vi "Memory Throughput Test PXIe-796XR (FPGA).vi"() -> ()   [LabVIEW 2013]
doc: "This test writes to and reads from external memory at maximum data rates and reports the total measured throughput. Varying the write and read grant time will directly affect the memory efficiency. The larger the grant time, then the larger the througput, and the lower the grant time, then the lower the throughput.\n\nDuring reads, the data is validated against an expected pattern. Failures will cause \"Read Data Error?\" to illuminate. To avoid read data errors, a full iteration of memory writes must be completed before starting the memory reads."
uses:
  <vilib>/Platform/TimedLoop/XDataNode/timing_clust.ctl
  <vilib>/Platform/TimedLoop/XDataNode/nitl_modes.ctl
  <vilib>/Platform/TimedLoop/XDataNode/wakeup.ctl
  DRAMElemReaderState.ctl
  Read Request Command.ctl
  <vilib>/rvi/Emulation/niFpgaSctlEmulationGetInTimedLoop.vi
  <vilib>/rvi/Emulation/niFpgaEmulationReportErrorSimple.vi
  <vilib>/rvi/Emulation/niFpgaGetClockAttributes.vi
  <vilib>/rvi/Emulation/niFpgaCriticalErrorInLSC.vi
  <vilib>/rvi/FIFO/Fifo_Resource/nirvififoEmulationWriteFpgaImpl.vi
  <vilib>/rvi/DataTransferAndStorage/Container/Common/niFpgaContainerGetUniqueNameForEmu.vi
  <vilib>/rvi/FIFO/Fifo_Resource/nirvififoEmulationReadFpgaImpl.vi
  <vilib>/rvi/Memory/Memory_Emulation/niFpgaMemoryEmulationReadFromVariant.vi
  <vilib>/rvi/Memory/Memory_Emulation/niFpgaMemoryFastEmulationDramWriteAndRequestData.vi
  <vilib>/rvi/Memory/Memory_Emulation/niFpgaMemoryEmulationDramWriteAndRequestData.vi
  <vilib>/rvi/Memory/Memory_Emulation/niFpgaMemoryEmulationWriteToVariant.vi
  <vilib>/Platform/TimedLoop/XDataNode/XDataNode.xnode
  <vilib>/rvi/DataTransferAndStorage/Container/XNode/niFpgaContainer.xnode
  <vilib>/rvi/FIFO/Fifo_Resource/nirvififoEmulationWrite.vi
  <vilib>/rvi/FIFO/Fifo_Resource/nirvififoEmulationRead.vi
  <vilib>/rvi/Memory/Memory_Emulation/niFpgaMemoryEmulationDramRetrieveData.vi
  <vilib>/Platform/TimedLoop/XDataNode/XDNodeRunTimeDep.lvlib
panel:
  in  "Write Req Grant Time (Bank 1)":u16=1000 caption="Write Req Grant Time (clocks)"
  in  "Read Req Grant Time (Bank 1)":u16=1000 caption="Read Req Grant Time (clocks)"
  in  "Read Req Grant Time (Bank 0)":u16=1000 caption="Read Req Grant Time (clocks)"
  in  "Write Req Grant Time (Bank 0)":u16=1000 caption="Write Req Grant Time (clocks)"
  out "Current Write Data Lower (Bank 0)":u64 caption="Current Write Data Lower" format="%.0x"
  out "Current Write Data Upper (Bank 0)":u64 caption="Current Write Data Upper" format="%.0x"
  out "Current Write Data Lower (Bank 1)":u64 caption="Current Write Data Lower" format="%.0x"
  out "Current Read Data Lower (Bank 1)":u64 caption="Current Read Data Lower" format="%.0x"
  out "Current Read Data Lower (Bank 0)":u64 caption="Current Read Data Lower" format="%.0x"
  out "Current Write Data Upper (Bank 1)":u64 caption="Current Write Data Upper" format="%.0x"
  out "Current Write Address (Bank 1)":u32 caption="Current Write Address" format="%.0x"
  in  "Enable Writes? (Bank 1)":bool=TRUE caption="Enable Writes?"
  out "Write Throughput (bytes/sec) (Bank 1)":u32 caption="Write Throughput (bytes/sec)" format="%.2e"
  out "Read FIFO Overflow? (Bank 1)":bool caption="Read FIFO Overflow?"
  out "Read Data Error? (Bank 1)":bool caption="Read Data Error?"
  out "Current Read Data Upper (Bank 1)":u64 caption="Current Read Data Upper" format="%.0x"
  out "Current Read Address (Bank 1)":u32 caption="Current Read Address" format="%.0x"
  in  "Enable Reads? (Bank 1)":bool caption="Enable Reads?"
  out "Read Throughput (bytes/sec) (Bank 1)":u32 caption="Read Throughput (bytes/sec)" format="%.2e"
  in  "DRAM Size (elements) (Bank 1)":u32=16777216 caption="DRAM Size (elements)"
  out "Read Data Error? (Bank 0)":bool caption="Read Data Error?"
  out "Write Throughput (bytes/sec) (Bank 0)":u32 caption="Write Throughput (bytes/sec)" format="%.2e"
  out "Read Throughput (bytes/sec) (Bank 0)":u32 caption="Read Throughput (bytes/sec)" format="%.2e"
  in  "Enable Reads? (Bank 0)":bool caption="Enable Reads?"
  out "Read FIFO Overflow? (Bank 0)":bool caption="Read FIFO Overflow?"
  in  "Enable Writes? (Bank 0)":bool=TRUE caption="Enable Writes?"
  out "Current Read Data Upper (Bank 0)":u64 caption="Current Read Data Upper" format="%.0x"
  in  "DRAM Size (elements) (Bank 0)":u32=16777216 caption="DRAM Size (elements)"
  out "Current Read Address (Bank 0)":u32 caption="Current Read Address" format="%.0x"
  out "Current Write Address (Bank 0)":u32 caption="Current Write Address" format="%.0x"
  # "Bank 0"
  # "Bank 1"
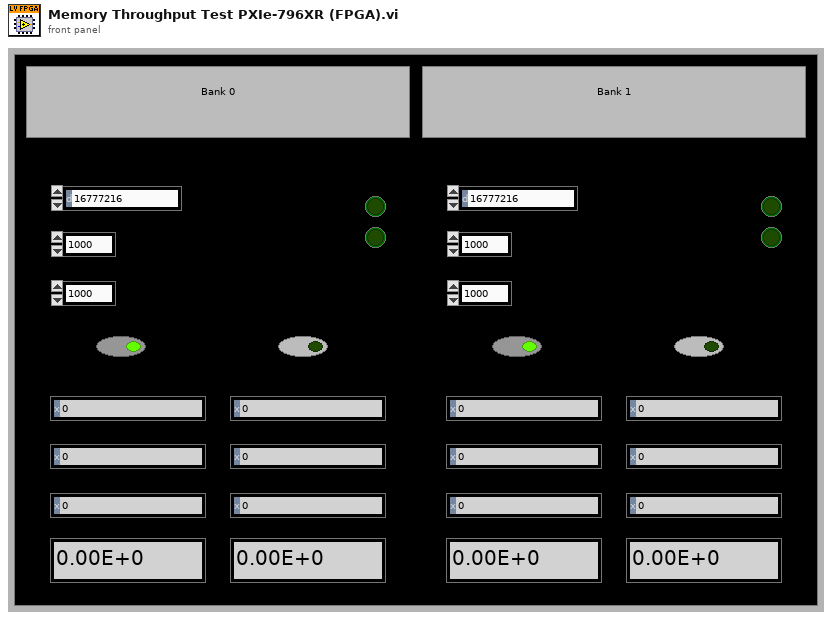
[diagram p1: front panel]
types:
  T1 = typedef "XDNodeRunTimeDep.lvlib/timing_clust.ctl" = cluster{"Expected End [f-1]":u64, "Actual End [f-1]":u64, "Finished Late? [f-1]":bool, "Expected End [i-1]":u64, "Actual End [i-1]":u64, "Finished Late? [i-1]":bool, "Expected Start [i]":u64, "Actual Start [i]":u64, "Expected Start [f]":u64, "Actual Start [f]":u64, "Source Name":string, "Structure Name":string, "Period":i64, "Deadline":i64, "Offset":i64, "Start":i64, "Priority":i32, "Timeout":i32, "Mode":T2, "Wakeup Reason":T3, "Error":errorcluster, "Source Type":string, "Secondary Source Type":string, "Global End Time":u64, "Global Start Time":u64, "Frame Duration":u64, "Iteration Duration":u64, "Assigned CPU":i32, "I/O Scan Engine Mode":u32}
  T2 = typedef "XDNodeRunTimeDep.lvlib/nitl_modes.ctl" = enum32{"No Change", "Process missed periods, maintain original phase", "Discard missed periods, maintain original phase", "Process missed periods, ignore original phase", "Discard missed periods, ignore original phase"}
  T3 = typedef "XDNodeRunTimeDep.lvlib/wakeup.ctl" = enum32{"Normal", "Aborted", "Asynchronous wakeup", "Timing source error", "Timed loop error", "Timeout"}
  T4 = cluster{"Address":u32, "Data":cluster{"Upper":u64, "Lower":u64}}
  T5 = typedef "DRAMElemReaderState.ctl" = enum16{"Start Read", "Wait for Read Complete"}
  T6 = typedef "Read Request Command.ctl" = cluster{"Address":u32, "Elements Remaining":u32, "Valid?":bool}
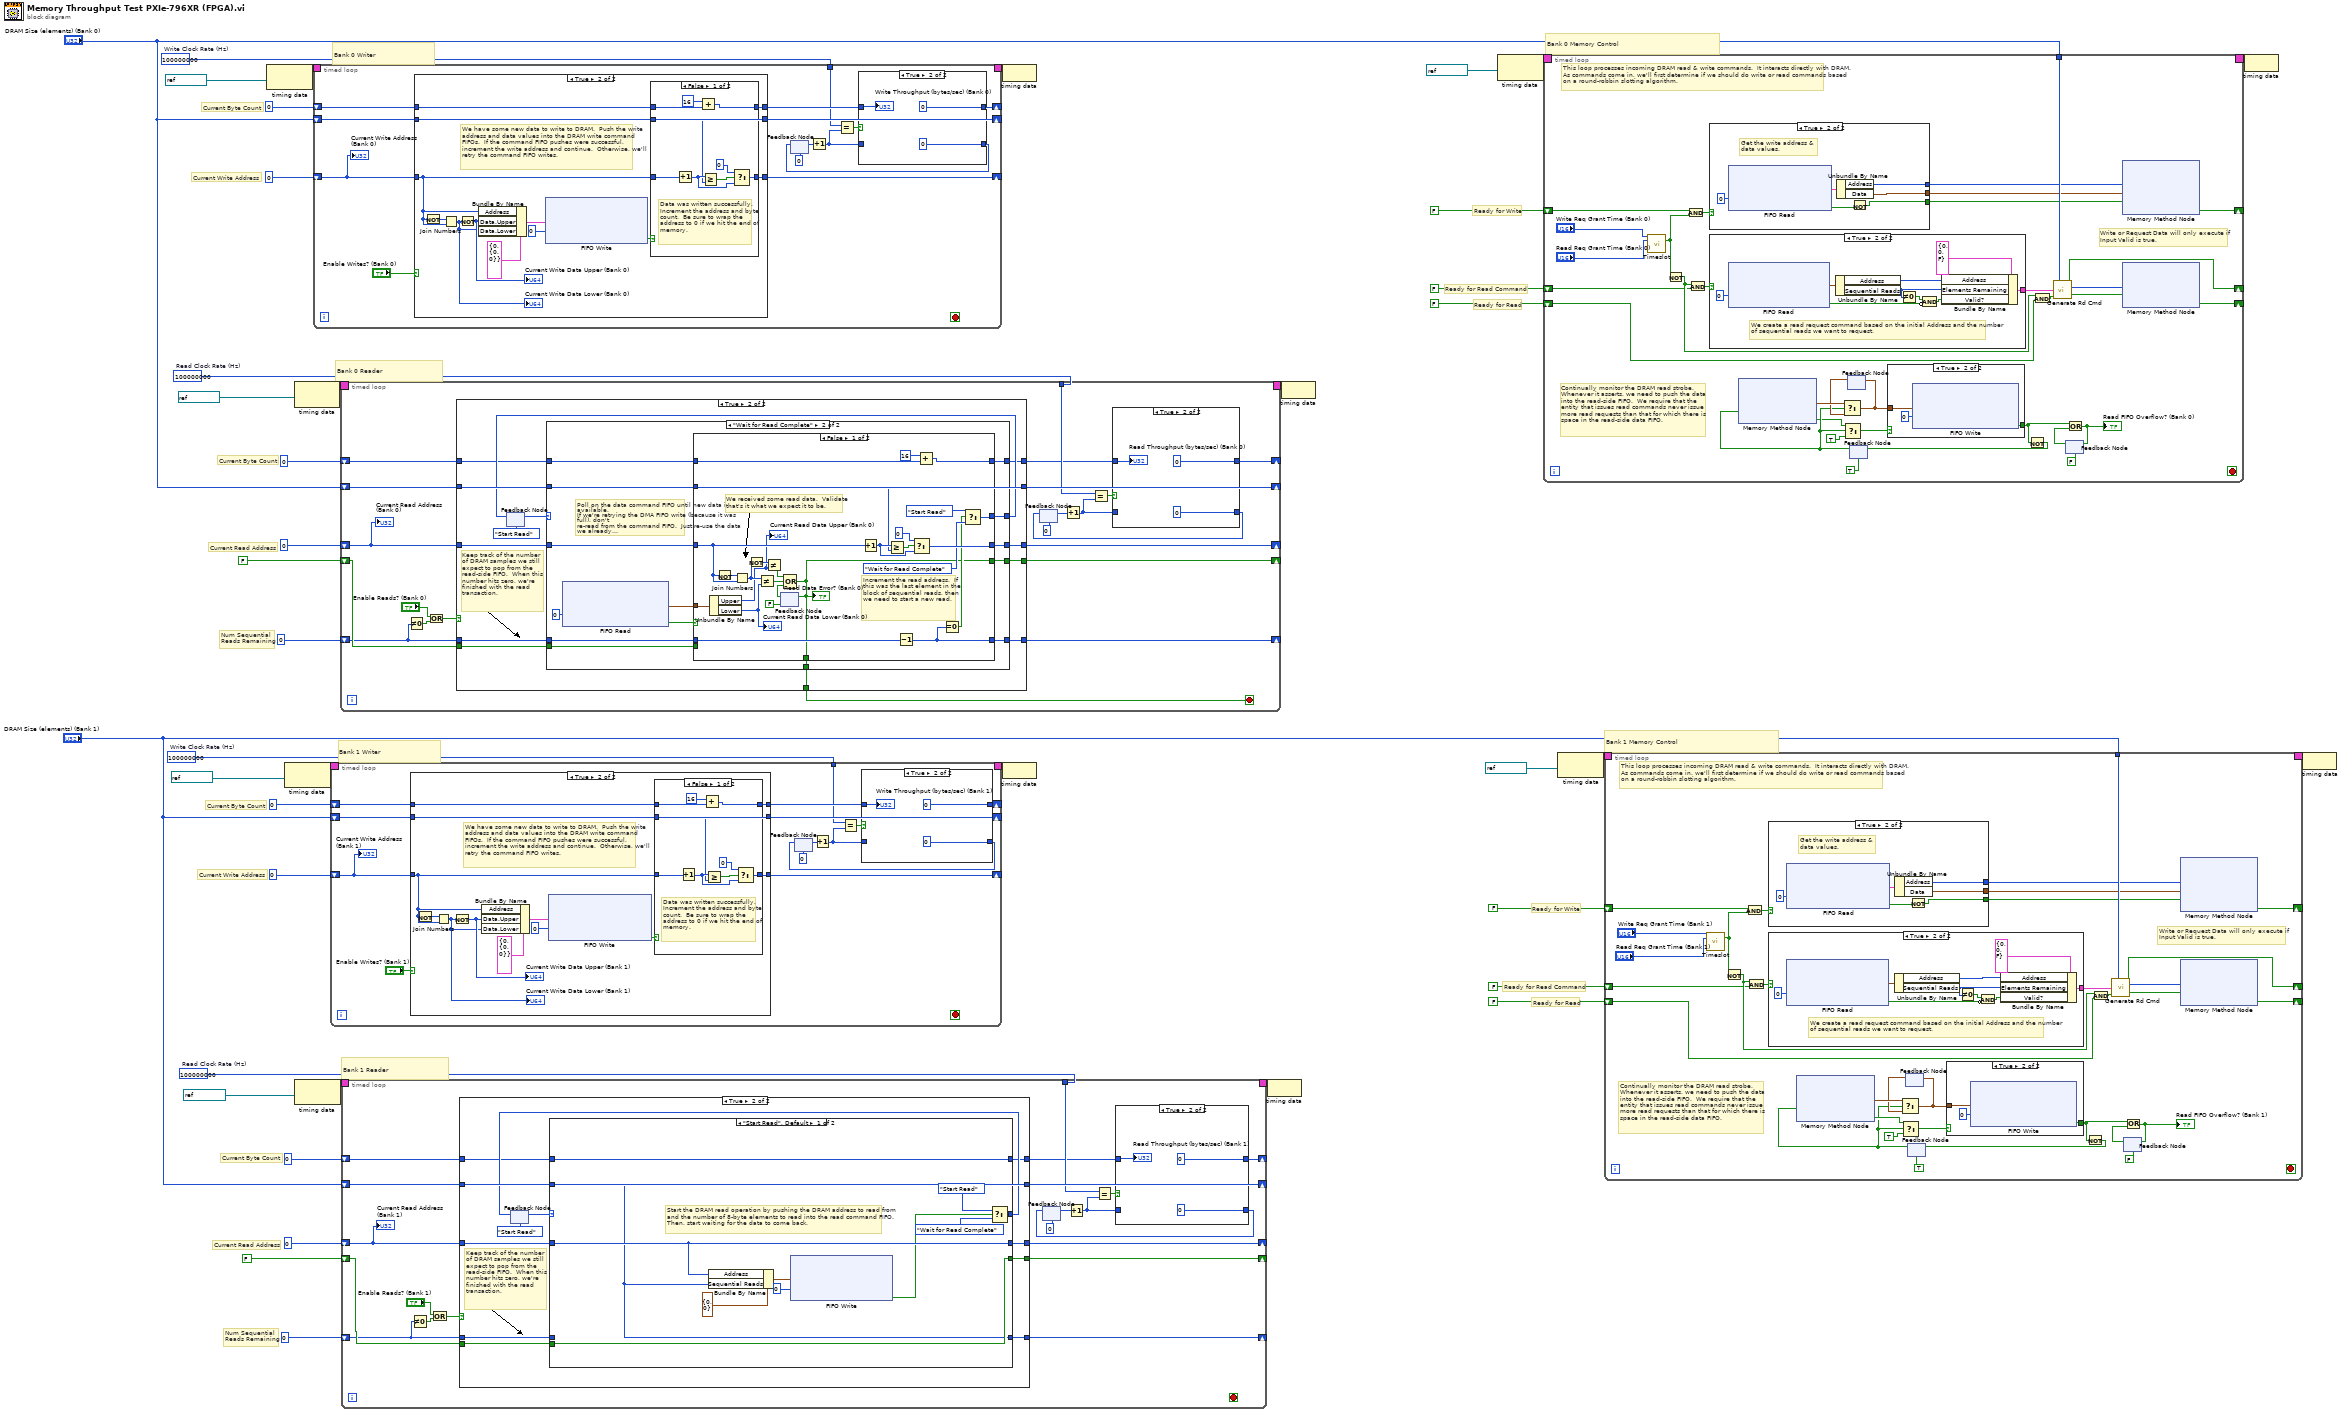
[diagram p0: block diagram]
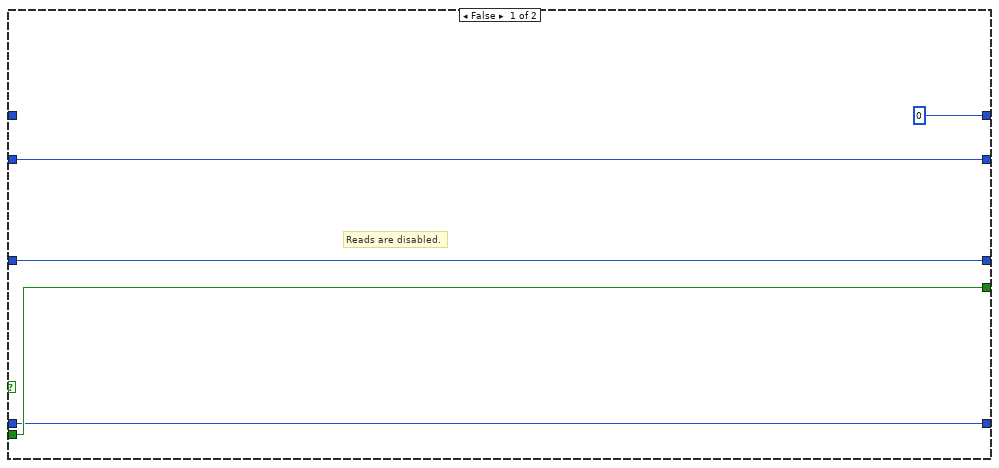
[diagram p3: hidden frame]
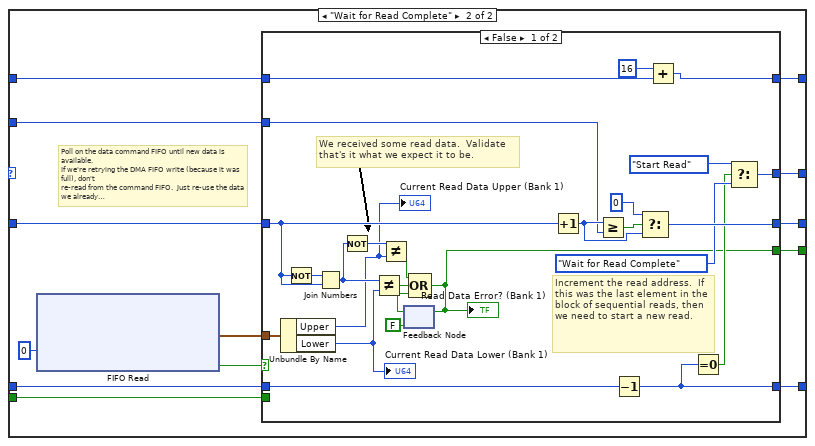
[diagram p4: hidden frame]
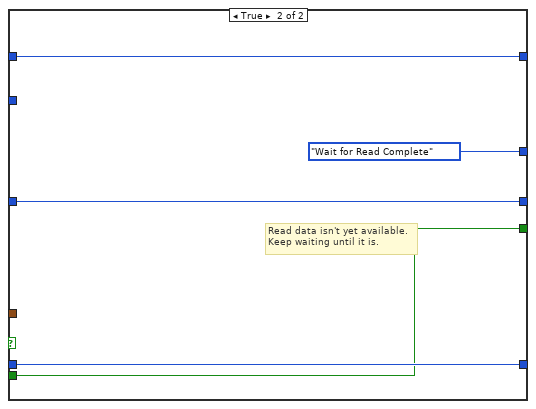
[diagram p5: hidden frame]
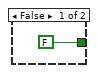
[diagram p6: hidden frame]
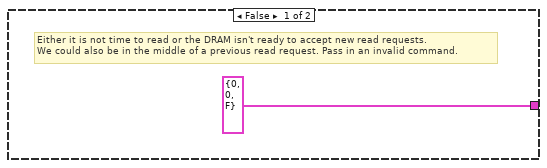
[diagram p7: hidden frame]
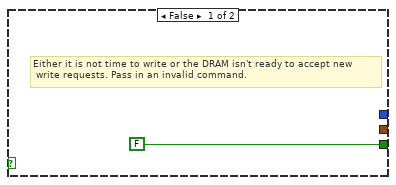
[diagram p8: hidden frame]
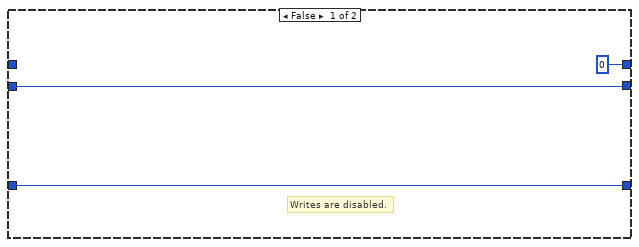
[diagram p10: hidden frame]
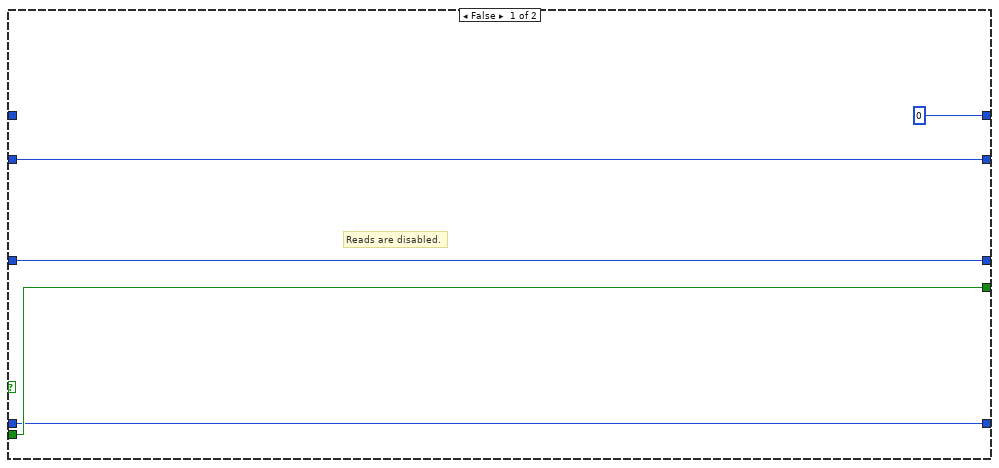
[diagram p13: hidden frame]
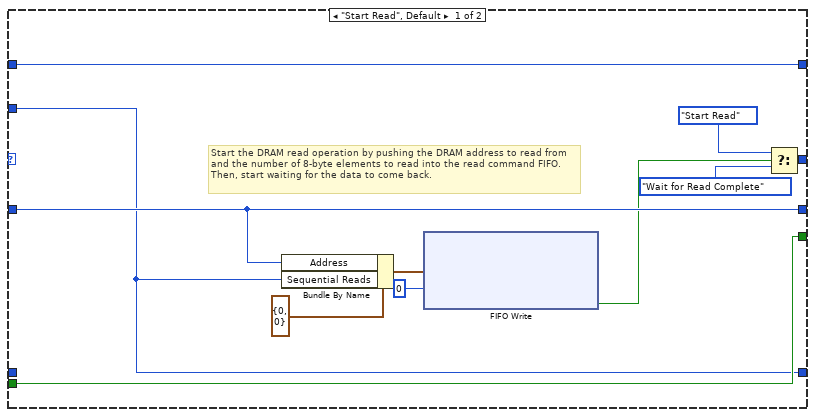
[diagram p14: hidden frame]
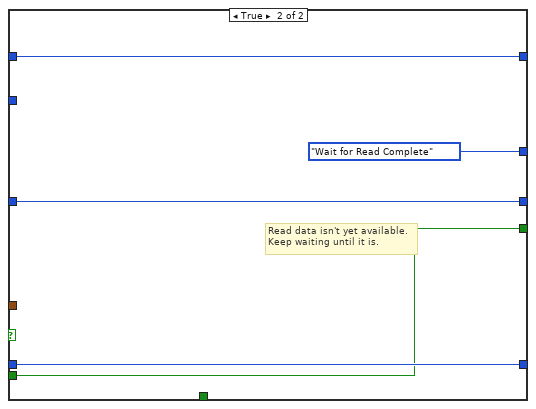
[diagram p15: hidden frame]
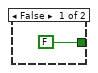
[diagram p16: hidden frame]
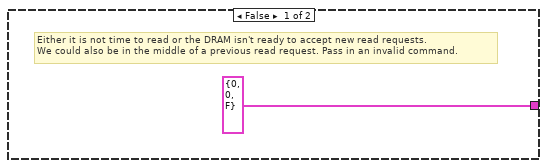
[diagram p17: hidden frame]
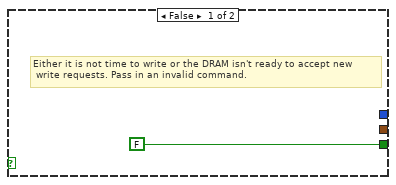
[diagram p18: hidden frame]
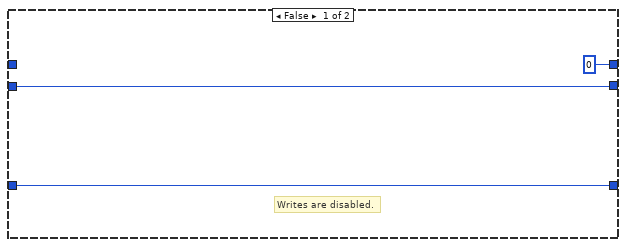
[diagram p20: hidden frame]
diagram:
  w3 = u32 100000000  # Read Clock Rate (Hz)
  w10 = u32 100000000  # Write Clock Rate (Hz)
  w4 = u32 100000000  # Read Clock Rate (Hz)
  w23 = u32 100000000  # Write Clock Rate (Hz)
  # "Ready for Read Command"
  # "Ready for Write"
  # "Ready for Read"
  # "Num Sequential\nReads Remaining"
  # "Bank 1 Memory Control"
  # "Bank 1 Reader"
  # "Bank 1 Writer"
  # "Current Byte Count"
  # "Current Byte Count"
  # "Current Read Address"
  # "Current Write Address"
  # "Ready for Read Command"
  # "Ready for Write"
  # "Ready for Read"
  # "Num Sequential\nReads Remaining"
  # "Bank 0 Memory Control"
  # "Bank 0 Reader"
  # "Bank 0 Writer"
  # "Current Byte Count"
  # "Current Byte Count"
  # "Current Read Address"
  # "Current Write Address"
  n1 = node-c288(refnum<k21> "100MHz" ("Source Name")) -> (w42:T1)
  n2 = node-c288(refnum<k21> "100MHz" ("Source Name")) -> (w36:T1)
  n3 = node-c288(refnum<k21> "100MHz" ("Source Name")) -> (w38:T1)
  n4 = node-c288(refnum<k21> "100MHz" ("Source Name")) -> (w32:T1)
  n5 = timed-loop {
    timing: w42 -> [_]
    timing-out: [_] -> w41
    shift-right: [w56] -> _
    shift-left: u32 0 -> [w43]
    shift-right: [w54] -> _
    shift-left: "DRAM Size (elements) (Bank 0)" -> [w55]
    shift-right: [w52] -> _
    shift-left: u32 0 -> [w53]
    tunnel: w23 -> [w45]
    stop <- _ stop-if-true
    n6 = case shown="True" "Enable Writes? (Bank 0)" {
      tunnel: w43 -> [w62 w67]
      tunnel: [w62 w76] -> w56
      tunnel: w55 -> [w63 w75]
      tunnel: [w63 w75] -> w54
      tunnel: w53 -> [_ w72]
      tunnel: [u32 0 w71] -> w51
      frame False {
        # "Writes are disabled."
      }
      frame True {
        # "We have some new data to write to DRAM.  Push the write address and data values into the DRAM write command FIFOs.  If the command FIFO pushes were successful, increment the write address and continue.  Otherwise, we'll retry the command FIFO writes."
        n7 = Not(x=w67) -> (.not. x?=w73:u32)
        n8 = Join Numbers(hi=w73, lo=w67) -> ((hi.lo)=w65:u64)
        "Current Write Data Lower (Bank 0)" <- w65
        n9 = Not(x=w65) -> (.not. x?=w66:u64)
        "Current Write Data Upper (Bank 0)" <- w66
        n10 = Bundle By Name(cluster=T4 {"Address"=0, "Data"={"Upper"=0, "Lower"=0}} ("Element"), "Address"=w67, "Data.Upper"=w66, "Data.Lower"=w65) -> (w68:T4)
        n11 = xnode ("FIFO Write")("Element"=w68, "Timeout"=0) -> ("Timed Out?"=w70:bool)  [unwired: 1 in, 1 out]
        n12 = case shown="False" w70 {
          tunnel: w75 -> [w77 _]
          tunnel: [w82 w87] -> w76
          tunnel: w67 -> [w81 w87]
          tunnel: w72 -> [w80 w86]
          tunnel: [w78 w86] -> w71
          frame False {
            # "Data was written successfully.  Increment the address and byte count.  Be sure to wrap the address to 0 if we hit the end of memory."
            n13 = Increment(x=w81) -> (x+1=w83:u32)
            n14 = Add(x=u32 16, y=w80) -> (x+y=w78:u32)
            n15 = Greater Or Equal?(x=w83, y=w77) -> (x >= y?=w85:bool)
            n16 = Select(t=u32 0, s=w85, f=w83) -> (s? t:f=w82:u32)
          }
          frame True {
          }
        }
      }
    }
    n17 = feedback #1(u32 0) -> (w50:u32)
    n18 = Increment(x=w50) -> (x+1=w46:u32)
    n19 = Equal?(x=w45, y=w46) -> (x = y?=w48:bool)
    n20 = case shown="True" w48 {
      tunnel: w46 -> [w58 _]
      tunnel: [w58 u32 0] -> w47
      tunnel: w51 -> [w57 w59]
      tunnel: [w57 u32 0] -> w52
      frame False {
      }
      frame True {
        "Write Throughput (bytes/sec) (Bank 0)" <- w59
      }
    }
    n21 = feedback-in #1(w47) -> ()
    "Current Write Address (Bank 0)" <- w43
  }
  n22 = timed-loop {
    timing: w36 -> [_]
    timing-out: [_] -> w35
    shift-right: [w103] -> _
    shift-left: u32 0 -> [w91]
    shift-right: [w101] -> _
    shift-left: "DRAM Size (elements) (Bank 1)" -> [w102]
    shift-right: [w99] -> _
    shift-left: u32 0 -> [w100]
    tunnel: w10 -> [w92]
    stop <- _ stop-if-true
    n23 = case shown="True" "Enable Writes? (Bank 1)" {
      tunnel: w91 -> [w109 w117]
      tunnel: [w109 w123] -> w103
      tunnel: w102 -> [w110 w122]
      tunnel: [w110 w122] -> w101
      tunnel: w100 -> [_ w119]
      tunnel: [u32 0 w118] -> w98
      frame False {
        # "Writes are disabled."
      }
      frame True {
        # "We have some new data to write to DRAM.  Push the write address and data values into the DRAM write command FIFOs.  If the command FIFO pushes were successful, increment the write address and continue.  Otherwise, we'll retry the command FIFO writes."
        n24 = Not(x=w117) -> (.not. x?=w120:u32)
        n25 = Join Numbers(hi=w120, lo=w117) -> ((hi.lo)=w112:u64)
        "Current Write Data Lower (Bank 1)" <- w112
        n26 = Not(x=w112) -> (.not. x?=w113:u64)
        "Current Write Data Upper (Bank 1)" <- w113
        n27 = Bundle By Name(cluster=T4 {"Address"=0, "Data"={"Upper"=0, "Lower"=0}} ("Element"), "Address"=w117, "Data.Upper"=w113, "Data.Lower"=w112) -> (w114:T4)
        n28 = xnode ("FIFO Write")("Element"=w114, "Timeout"=0) -> ("Timed Out?"=w116:bool)  [unwired: 1 in, 1 out]
        n29 = case shown="False" w116 {
          tunnel: w122 -> [w124 _]
          tunnel: [w129 w134] -> w123
          tunnel: w117 -> [w128 w134]
          tunnel: w119 -> [w127 w133]
          tunnel: [w125 w133] -> w118
          frame False {
            # "Data was written successfully.  Increment the address and byte count.  Be sure to wrap the address to 0 if we hit the end of memory."
            n30 = Increment(x=w128) -> (x+1=w130:u32)
            n31 = Add(x=u32 16, y=w127) -> (x+y=w125:u32)
            n32 = Greater Or Equal?(x=w130, y=w124) -> (x >= y?=w132:bool)
            n33 = Select(t=u32 0, s=w132, f=w130) -> (s? t:f=w129:u32)
          }
          frame True {
          }
        }
      }
    }
    n34 = feedback #2(u32 0) -> (w97:u32)
    n35 = Increment(x=w97) -> (x+1=w93:u32)
    n36 = Equal?(x=w92, y=w93) -> (x = y?=w95:bool)
    n37 = case shown="True" w95 {
      tunnel: w93 -> [w105 _]
      tunnel: [w105 u32 0] -> w94
      tunnel: w98 -> [w104 w106]
      tunnel: [w104 u32 0] -> w99
      frame False {
      }
      frame True {
        "Write Throughput (bytes/sec) (Bank 1)" <- w106
      }
    }
    n38 = feedback-in #2(w94) -> ()
    "Current Write Address (Bank 1)" <- w91
  }
  n39 = timed-loop {
    timing: w38 -> [_]
    timing-out: [_] -> w37
    shift-right: [w157] -> _
    shift-left: u32 0 -> [w139]
    shift-right: [w155] -> _
    shift-left: "DRAM Size (elements) (Bank 0)" -> [w156]
    shift-right: [w153] -> _
    shift-left: u32 0 -> [w154]
    tunnel: w4 -> [w152]
    shift-right: [w151] -> _
    shift-left: u32 0 -> [w141]
    shift-right: [w144] -> _
    shift-left: FALSE -> [w143]
    stop <- w137 stop-if-true
    n40 = Not Equal To 0?(x=w141) -> (x != 0?=w142:bool)
    n41 = Or(x="Enable Reads? (Bank 0)", y=w142) -> (x .or. y?=w140:bool)
    n42 = case shown="True" w140 {
      tunnel: w139 -> [w165 w179]
      tunnel: [w165 w180] -> w157
      tunnel: w156 -> [w164 w178]
      tunnel: [w164 w178] -> w155
      tunnel: w154 -> [_ w174]
      tunnel: [u32 0 w173] -> w146
      tunnel: [w163 w172] -> w151
      tunnel: w141 -> [w163 w171]
      tunnel: [w166 w170] -> w144
      tunnel: w143 -> [w166 w169]
      tunnel: [_ w168] -> w137
      frame False {
        # "Reads are disabled."
      }
      frame True {
        # "Keep track of the number\nof DRAM samples we still\nexpect to pop from the\nread-side FIFO.  When this\nnumber hits zero, we're\nfinished with the read\ntransaction."
        n43 = feedback #3(DRAMElemReaderState."Start Read") -> (w175:T5)
        n44 = case shown="\"Wait for Read Complete\"" w175 {
          tunnel: [w184 w204] -> w176
          tunnel: w179 -> [w187 w196]
          tunnel: [w187 w205] -> w180
          tunnel: w178 -> [w181 w202]
          tunnel: w171 -> [_ w200]
          tunnel: [w181 w201] -> w172
          tunnel: w174 -> [w190 w198]
          tunnel: [w190 w197] -> w173
          tunnel: [w183 w194] -> w170
          tunnel: w169 -> [w183 w193]
          tunnel: [_ w192] -> w168
          frame "Start Read", Default {
            # "Start the DRAM read operation by pushing the DRAM address to read from and the number of 8-byte elements to read into the read command FIFO.  Then, start waiting for the data to come back."
            n45 = Bundle By Name(cluster=cluster{"Address":u32, "Sequential Reads":u32} {"Address"=0, "Sequential Reads"=0} ("Element"), "Address"=w187, "Sequential Reads"=w181) -> (w189:cluster{"Address":u32, "Sequential Reads":u32})
            n46 = xnode ("FIFO Write")("Element"=w189, "Timeout"=0) -> ("Timed Out?"=w186:bool)  [unwired: 1 in, 1 out]
            n47 = Select(t=DRAMElemReaderState."Start Read", s=w186, f=DRAMElemReaderState."Wait for Read Complete") -> (s? t:f=w184:T5)
          }
          frame "Wait for Read Complete" {
            # "Poll on the data command FIFO until new data is available.\nIf we're retrying the DMA FIFO write (because it was full), don't\nre-read from the command FIFO.  Just re-use the data we already\nread."
            n48 = xnode ("FIFO Read")("Timeout"=0) -> ("Element"=w195:cluster{"Upper":u64, "Lower":u64}, "Timed Out?"=w203:bool)  [unwired: 1 in, 1 out]
            n49 = case shown="False" w203 {
              tunnel: w196 -> [w218 w236]
              tunnel: [w230 w236] -> w205
              tunnel: [w231 DRAMElemReaderState."Wait for Read Complete"] -> w204
              tunnel: w195 -> [w212 _]
              tunnel: w202 -> [w216 _]
              tunnel: w200 -> [w229 w235]
              tunnel: [w215 w235] -> w201
              tunnel: w198 -> [w223 w234]
              tunnel: [w221 w234] -> w197
              tunnel: [w206 w232] -> w194
              tunnel: w193 -> [_ w232]
              tunnel: [w206 _] -> w192
              frame False {
                # "Increment the read address.  If this was the last element in the block of sequential reads, then we need to start a new read."
                # "We received some read data.  Validate\nthat's it what we expect it to be."
                n50 = Unbundle By Name(w212) -> ("Upper"=w207:u64, "Lower"=w208:u64)
                "Current Read Data Upper (Bank 0)" <- w207
                "Current Read Data Lower (Bank 0)" <- w208
                n51 = Not(x=w218) -> (.not. x?=w217:u32)
                n52 = Join Numbers(hi=w217, lo=w218) -> ((hi.lo)=w211:u64)
                n53 = Not(x=w211) -> (.not. x?=w209:u64)
                n54 = Not Equal?(x=w211, y=w208) -> (x != y?=w214:bool)
                n55 = Not Equal?(x=w209, y=w207) -> (x != y?=w210:bool)
                n56 = feedback #4(FALSE) -> (w220:bool)
                n57 = Compound Arithmetic op=OR(w210, w214, w220) -> (w206:bool)
                "Read Data Error? (Bank 0)" <- w206
                n58 = feedback-in #4(w206) -> ()
                n59 = Increment(x=w218) -> (x+1=w227:u32)
                n60 = Greater Or Equal?(x=w227, y=w216) -> (x >= y?=w213:bool)
                n61 = Decrement(x=w229) -> (x-1=w215:u32)
                n62 = Select(t=u32 0, s=w213, f=w227) -> (s? t:f=w230:u32)
                n63 = Add(x=u32 16, y=w223) -> (x+y=w221:u32)
                n64 = Equal To 0?(x=w215) -> (x = 0?=w224:bool)
                n65 = Select(t=DRAMElemReaderState."Start Read", s=w224, f=DRAMElemReaderState."Wait for Read Complete") -> (s? t:f=w231:T5)
              }
              frame True {
                # "Read data isn't yet available.\nKeep waiting until it is."
              }
            }
          }
        }
        n66 = feedback-in #3(w176) -> ()
      }
    }
    n67 = feedback #5(u32 0) -> (w149:u32)
    n68 = Increment(x=w149) -> (x+1=w147:u32)
    n69 = Equal?(x=w152, y=w147) -> (x = y?=w148:bool)
    n70 = case shown="True" w148 {
      tunnel: w147 -> [w159 _]
      tunnel: [w159 u32 0] -> w145
      tunnel: w146 -> [w158 w160]
      tunnel: [w158 u32 0] -> w153
      frame False {
      }
      frame True {
        "Read Throughput (bytes/sec) (Bank 0)" <- w160
      }
    }
    n71 = feedback-in #5(w145) -> ()
    "Current Read Address (Bank 0)" <- w139
  }
  n72 = timed-loop {
    timing: w32 -> [_]
    timing-out: [_] -> w31
    shift-right: [w258] -> _
    shift-left: u32 0 -> [w240]
    shift-right: [w256] -> _
    shift-left: "DRAM Size (elements) (Bank 1)" -> [w257]
    shift-right: [w254] -> _
    shift-left: u32 0 -> [w255]
    tunnel: w3 -> [w253]
    shift-right: [w252] -> _
    shift-left: u32 0 -> [w242]
    shift-right: [w245] -> _
    shift-left: FALSE -> [w244]
    stop <- _ stop-if-true
    n73 = Not Equal To 0?(x=w242) -> (x != 0?=w243:bool)
    n74 = Or(x="Enable Reads? (Bank 1)", y=w243) -> (x .or. y?=w241:bool)
    n75 = case shown="True" w241 {
      tunnel: w240 -> [w266 w279]
      tunnel: [w266 w280] -> w258
      tunnel: w257 -> [w265 w278]
      tunnel: [w265 w278] -> w256
      tunnel: w255 -> [_ w274]
      tunnel: [u32 0 w273] -> w247
      tunnel: [w264 w272] -> w252
      tunnel: w242 -> [w264 w271]
      tunnel: [w267 w270] -> w245
      tunnel: w244 -> [w267 w269]
      frame False {
        # "Reads are disabled."
      }
      frame True {
        # "Keep track of the number\nof DRAM samples we still\nexpect to pop from the\nread-side FIFO.  When this\nnumber hits zero, we're\nfinished with the read\ntransaction."
        n76 = feedback #6(DRAMElemReaderState."Start Read") -> (w275:T5)
        n77 = case shown="\"Start Read\", Default" w275 {
          tunnel: [w284 w303] -> w276
          tunnel: w279 -> [w287 w295]
          tunnel: [w287 w304] -> w280
          tunnel: w278 -> [w281 w301]
          tunnel: w271 -> [_ w299]
          tunnel: [w281 w300] -> w272
          tunnel: w274 -> [w290 w297]
          tunnel: [w290 w296] -> w273
          tunnel: [w283 w293] -> w270
          tunnel: w269 -> [w283 w292]
          frame "Start Read", Default {
            # "Start the DRAM read operation by pushing the DRAM address to read from and the number of 8-byte elements to read into the read command FIFO.  Then, start waiting for the data to come back."
            n78 = Bundle By Name(cluster=cluster{"Address":u32, "Sequential Reads":u32} {"Address"=0, "Sequential Reads"=0} ("Element"), "Address"=w287, "Sequential Reads"=w281) -> (w289:cluster{"Address":u32, "Sequential Reads":u32})
            n79 = xnode ("FIFO Write")("Element"=w289, "Timeout"=0) -> ("Timed Out?"=w286:bool)  [unwired: 1 in, 1 out]
            n80 = Select(t=DRAMElemReaderState."Start Read", s=w286, f=DRAMElemReaderState."Wait for Read Complete") -> (s? t:f=w284:T5)
          }
          frame "Wait for Read Complete" {
            # "Poll on the data command FIFO until new data is available.\nIf we're retrying the DMA FIFO write (because it was full), don't\nre-read from the command FIFO.  Just re-use the data we already\nread."
            n81 = xnode ("FIFO Read")("Timeout"=0) -> ("Element"=w294:cluster{"Upper":u64, "Lower":u64}, "Timed Out?"=w302:bool)  [unwired: 1 in, 1 out]
            n82 = case shown="False" w302 {
              tunnel: w295 -> [w307 w335]
              tunnel: [w329 w335] -> w304
              tunnel: [w330 DRAMElemReaderState."Wait for Read Complete"] -> w303
              tunnel: w294 -> [w311 _]
              tunnel: w301 -> [w316 _]
              tunnel: w299 -> [w328 w334]
              tunnel: [w315 w334] -> w300
              tunnel: w297 -> [w322 w333]
              tunnel: [w320 w333] -> w296
              tunnel: [w312 w331] -> w293
              tunnel: w292 -> [_ w331]
              frame False {
                # "Increment the read address.  If this was the last element in the block of sequential reads, then we need to start a new read."
                # "We received some read data.  Validate\nthat's it what we expect it to be."
                n83 = Unbundle By Name(w311) -> ("Upper"=w306:u64, "Lower"=w305:u64)
                "Current Read Data Lower (Bank 1)" <- w305
                "Current Read Data Upper (Bank 1)" <- w306
                n84 = Not(x=w307) -> (.not. x?=w317:u32)
                n85 = Join Numbers(hi=w317, lo=w307) -> ((hi.lo)=w310:u64)
                n86 = Not(x=w310) -> (.not. x?=w309:u64)
                n87 = Not Equal?(x=w310, y=w305) -> (x != y?=w314:bool)
                n88 = Not Equal?(x=w309, y=w306) -> (x != y?=w308:bool)
                n89 = feedback #7(FALSE) -> (w319:bool)
                n90 = Compound Arithmetic op=OR(w308, w314, w319) -> (w312:bool)
                "Read Data Error? (Bank 1)" <- w312
                n91 = feedback-in #7(w312) -> ()
                n92 = Increment(x=w307) -> (x+1=w326:u32)
                n93 = Greater Or Equal?(x=w326, y=w316) -> (x >= y?=w313:bool)
                n94 = Decrement(x=w328) -> (x-1=w315:u32)
                n95 = Select(t=u32 0, s=w313, f=w326) -> (s? t:f=w329:u32)
                n96 = Add(x=u32 16, y=w322) -> (x+y=w320:u32)
                n97 = Equal To 0?(x=w315) -> (x = 0?=w323:bool)
                n98 = Select(t=DRAMElemReaderState."Start Read", s=w323, f=DRAMElemReaderState."Wait for Read Complete") -> (s? t:f=w330:T5)
              }
              frame True {
                # "Read data isn't yet available.\nKeep waiting until it is."
              }
            }
          }
        }
        n99 = feedback-in #6(w276) -> ()
      }
    }
    n100 = feedback #8(u32 0) -> (w250:u32)
    n101 = Increment(x=w250) -> (x+1=w248:u32)
    n102 = Equal?(x=w253, y=w248) -> (x = y?=w249:bool)
    n103 = case shown="True" w249 {
      tunnel: w248 -> [w260 _]
      tunnel: [w260 u32 0] -> w246
      tunnel: w247 -> [w259 w261]
      tunnel: [w259 u32 0] -> w254
      frame False {
      }
      frame True {
        "Read Throughput (bytes/sec) (Bank 1)" <- w261
      }
    }
    n104 = feedback-in #8(w246) -> ()
    "Current Read Address (Bank 1)" <- w240
  }
  n105 = node-c288(w41) -> ()
  n106 = node-c288(w35) -> ()
  n107 = node-c288(w31) -> ()
  n108 = node-c288(w37) -> ()
  n109 = node-c288(refnum<k21> "100MHz" ("Source Name")) -> (w40:T1)
  n110 = timed-loop {
    timing: w40 -> [_]
    timing-out: [_] -> w39
    tunnel: "DRAM Size (elements) (Bank 0)" -> [w361]
    shift-right: [w368] -> _
    shift-left: FALSE ("Ready for Input") -> [w342]
    shift-right: [w367] -> _
    shift-left: FALSE ("Ready for Input") -> [w365]
    shift-right: [w360] -> _
    shift-left: FALSE ("ready for input") -> [w357]
    stop <- _ stop-if-true
    # "Write or Request Data will only execute if \nInput Valid is true."
    # "Continually monitor the DRAM read strobe.\nWhenever it asserts, we need to push the data\ninto the read-side FIFO.  We require that the\nentity that issues read commands never issue\nmore read requests than that for which there is\nspace in the read-side data FIFO."
    # "This loop processes incoming DRAM read & write commands.  It interacts directly with DRAM.  \nAs commands come in, we'll first determine if we should do write or read commands based \non a round-robbin slotting algorithm."
    n111 = call "Timeslot.vi"("Write Req Grant Time (clocks)"="Write Req Grant Time (Bank 0)", "Read Req Grant Time (clocks)"="Read Req Grant Time (Bank 0)") -> ("Mux Select"=w364:bool)  [unwired: 13 in]
    n112 = Not(x=w364) -> (.not. x?=w358:bool)
    n113 = And(x=w365, y=w364) -> (x .and. y?=w366:bool)
    n114 = And(x=w358, y=w357) -> (x .and. y?=w363:bool)
    n115 = case shown="True" w366 {
      tunnel: [_ w388] -> w356
      tunnel: [_ w387] -> w355
      tunnel: [FALSE w386] -> w354
      frame False {
        # "Either it is not time to write or the DRAM isn't ready to accept new\n write requests. Pass in an invalid command."
      }
      frame True {
        # "Get the write address & data values."
        n116 = xnode ("FIFO Read")("Timeout"=0) -> ("Element"=w389:T4, "Timed Out?"=w390:bool)  [unwired: 1 in, 1 out]
        n117 = Unbundle By Name(w389) -> ("Address"=w388:u32, "Data"=w387:cluster{"Upper":u64, "Lower":u64})
        n118 = Not(x=w390) -> (.not. x?=w386:bool)
      }
    }
    n119 = case shown="True" w363 {
      tunnel: [T6 {"Address"=0, "Elements Remaining"=0, "Valid?"=FALSE} ("Read request") w376] -> w362
      frame False {
        # "Either it is not time to read or the DRAM isn't ready to accept new read requests.\nWe could also be in the middle of a previous read request. Pass in an invalid command."
      }
      frame True {
        # "We create a read request command based on the initial Address and the number of sequential reads we want to request."
        n120 = xnode ("FIFO Read")("Timeout"=0) -> ("Element"=w382:cluster{"Address":u32, "Sequential Reads":u32}, "Timed Out?"=w380:bool)  [unwired: 1 in, 1 out]
        n121 = Unbundle By Name(w382) -> ("Address"=w381:u32, "Sequential Reads"=w379:u32)
        n122 = Not Equal To 0?(x=w379) -> (x != 0?=w383:bool)
        n123 = Compound Arithmetic op=AND(w383, invert w380) -> (w378:bool)
        n124 = Bundle By Name(cluster=T6 {"Address"=0, "Elements Remaining"=0, "Valid?"=FALSE} ("Read request"), "Address"=w381, "Elements Remaining"=w379, "Valid?"=w378) -> (w376:T6)
      }
    }
    n125 = feedback #9() -> (w350:cluster{"Upper":u64, "Lower":u64})  [unwired: 1 in]
    n126 = feedback #10(TRUE) -> (w343:bool)
    n127 = xnode ("Memory Method Node")("Ready For Output"=w343) -> ("Data"=w351:cluster{"Upper":u64, "Lower":u64}, "Output Valid"=w338:bool)  [unwired: 1 in, 1 out]
    n128 = Select(t=w351, s=w343, f=w350) -> (s? t:f=w349:cluster{"Upper":u64, "Lower":u64})
    n129 = Select(t=w338, s=w343, f=TRUE) -> (s? t:f=w345:bool)
    n130 = feedback-in #9(w349) -> ()
    n131 = case shown="True" w345 {
      tunnel: [FALSE ("Timed Out?") w373] -> w348
      tunnel: w349 -> [_ w372]
      frame False {
      }
      frame True {
        n132 = xnode ("FIFO Write")("Element"=w372, "Timeout"=0) -> ("Timed Out?"=w373:bool)  [unwired: 1 in, 1 out]
      }
    }
    n133 = Not(x=w348) -> (.not. x?=w347:bool)
    n134 = feedback-in #10(w347) -> ()
    n135 = And(x=w358, y=w342) -> (x .and. y?=w359:bool)
    n136 = call "Generate Rd Cmd.vi"("Number of Elements"=w361, "next Read request"=w362, "Ready for Read"=w359) -> ("ready for input"=w360:bool, "Address"=w353:u32, "Valid?"=w352:bool)  [unwired: 10 in]
    n137 = feedback #11(FALSE) -> (w370:bool)
    n138 = Or(x=w348, y=w370) -> (x .or. y?=w341:bool)
    "Read FIFO Overflow? (Bank 0)" <- w341
    n139 = feedback-in #11(w341) -> ()
    n140 = xnode ("Memory Method Node")("Address"=w356, "Data"=w355, "Input Valid"=w354) -> ("Ready For Input"=w367:bool)  [unwired: 1 in, 1 out]
    n141 = xnode ("Memory Method Node")("Address"=w353, "Input Valid"=w352) -> ("Ready For Input"=w368:bool)  [unwired: 1 in, 1 out]
  }
  n142 = node-c288(refnum<k21> "100MHz" ("Source Name")) -> (w34:T1)
  n143 = timed-loop {
    timing: w34 -> [_]
    timing-out: [_] -> w33
    tunnel: "DRAM Size (elements) (Bank 1)" -> [w417]
    shift-right: [w424] -> _
    shift-left: FALSE ("Ready for Input") -> [w397]
    shift-right: [w423] -> _
    shift-left: FALSE ("Ready for Input") -> [w421]
    shift-right: [w416] -> _
    shift-left: FALSE ("ready for input") -> [w413]
    stop <- _ stop-if-true
    # "Write or Request Data will only execute if \nInput Valid is true."
    # "Continually monitor the DRAM read strobe.\nWhenever it asserts, we need to push the data\ninto the read-side FIFO.  We require that the\nentity that issues read commands never issue\nmore read requests than that for which there is\nspace in the read-side data FIFO."
    # "This loop processes incoming DRAM read & write commands.  It interacts directly with DRAM.  \nAs commands come in, we'll first determine if we should do write or read commands based \non a round-robbin slotting algorithm."
    n144 = call "Timeslot.vi"("Write Req Grant Time (clocks)"="Write Req Grant Time (Bank 1)", "Read Req Grant Time (clocks)"="Read Req Grant Time (Bank 1)") -> ("Mux Select"=w420:bool)  [unwired: 13 in]
    n145 = Not(x=w420) -> (.not. x?=w414:bool)
    n146 = And(x=w421, y=w420) -> (x .and. y?=w422:bool)
    n147 = And(x=w414, y=w413) -> (x .and. y?=w419:bool)
    n148 = case shown="True" w422 {
      tunnel: [_ w444] -> w412
      tunnel: [_ w443] -> w411
      tunnel: [FALSE w442] -> w410
      frame False {
        # "Either it is not time to write or the DRAM isn't ready to accept new\n write requests. Pass in an invalid command."
      }
      frame True {
        # "Get the write address & data values."
        n149 = xnode ("FIFO Read")("Timeout"=0) -> ("Element"=w445:T4, "Timed Out?"=w446:bool)  [unwired: 1 in, 1 out]
        n150 = Unbundle By Name(w445) -> ("Address"=w444:u32, "Data"=w443:cluster{"Upper":u64, "Lower":u64})
        n151 = Not(x=w446) -> (.not. x?=w442:bool)
      }
    }
    n152 = case shown="True" w419 {
      tunnel: [T6 {"Address"=0, "Elements Remaining"=0, "Valid?"=FALSE} ("Read request") w432] -> w418
      frame False {
        # "Either it is not time to read or the DRAM isn't ready to accept new read requests.\nWe could also be in the middle of a previous read request. Pass in an invalid command."
      }
      frame True {
        # "We create a read request command based on the initial Address and the number of sequential reads we want to request."
        n153 = xnode ("FIFO Read")("Timeout"=0) -> ("Element"=w438:cluster{"Address":u32, "Sequential Reads":u32}, "Timed Out?"=w436:bool)  [unwired: 1 in, 1 out]
        n154 = Unbundle By Name(w438) -> ("Address"=w437:u32, "Sequential Reads"=w435:u32)
        n155 = Not Equal To 0?(x=w435) -> (x != 0?=w439:bool)
        n156 = Compound Arithmetic op=AND(w439, invert w436) -> (w434:bool)
        n157 = Bundle By Name(cluster=T6 {"Address"=0, "Elements Remaining"=0, "Valid?"=FALSE} ("Read request"), "Address"=w437, "Elements Remaining"=w435, "Valid?"=w434) -> (w432:T6)
      }
    }
    n158 = feedback #12() -> (w406:cluster{"Upper":u64, "Lower":u64})  [unwired: 1 in]
    n159 = feedback #13(TRUE) -> (w398:bool)
    n160 = xnode ("Memory Method Node")("Ready For Output"=w398) -> ("Data"=w407:cluster{"Upper":u64, "Lower":u64}, "Output Valid"=w401:bool)  [unwired: 1 in, 1 out]
    n161 = Select(t=w407, s=w398, f=w406) -> (s? t:f=w405:cluster{"Upper":u64, "Lower":u64})
    n162 = Select(t=w401, s=w398, f=TRUE) -> (s? t:f=w400:bool)
    n163 = feedback-in #12(w405) -> ()
    n164 = case shown="True" w400 {
      tunnel: [FALSE ("Timed Out?") w429] -> w404
      tunnel: w405 -> [_ w428]
      frame False {
      }
      frame True {
        n165 = xnode ("FIFO Write")("Element"=w428, "Timeout"=0) -> ("Timed Out?"=w429:bool)  [unwired: 1 in, 1 out]
      }
    }
    n166 = Not(x=w404) -> (.not. x?=w403:bool)
    n167 = feedback-in #13(w403) -> ()
    n168 = And(x=w414, y=w397) -> (x .and. y?=w415:bool)
    n169 = call "Generate Rd Cmd.vi"("Number of Elements"=w417, "next Read request"=w418, "Ready for Read"=w415) -> ("ready for input"=w416:bool, "Address"=w409:u32, "Valid?"=w408:bool)  [unwired: 10 in]
    n170 = feedback #14(FALSE) -> (w426:bool)
    n171 = Or(x=w404, y=w426) -> (x .or. y?=w394:bool)
    "Read FIFO Overflow? (Bank 1)" <- w394
    n172 = feedback-in #14(w394) -> ()
    n173 = xnode ("Memory Method Node")("Address"=w412, "Data"=w411, "Input Valid"=w410) -> ("Ready For Input"=w423:bool)  [unwired: 1 in, 1 out]
    n174 = xnode ("Memory Method Node")("Address"=w409, "Input Valid"=w408) -> ("Ready For Input"=w424:bool)  [unwired: 1 in, 1 out]
  }
  n175 = node-c288(w39) -> ()
  n176 = node-c288(w33) -> ()
